vi "Sub_Initialize_LEMP_del.vi"(1 "Stiff":T2, 2 "Mass":T2) -> (0 "LEMP":T1)   [LabVIEW 2021]
uses:
  <vilib>/Analysis/Matrix/Datatypes/RealMatrix.ctl
  <vilib>/Analysis/Matrix/Numeric/Conversions/Matrix To Array - RM.vi
  <vilib>/Analysis/Matrix/NI_Matrix.lvlib
panel:
  # "Input"
  # "Output"
  # "This VI acquires the required input cluster for the Sub_online_LEMP_Update.vi, this VI calls on SciPy.linalg.eigh() due to issues with the standard \"General Eigenvalues and Eigenvectors.vi\" outputting inappropriately scaled eigenvectors for the LEMP. Additionally the Bitedness of this installation of LabVIEW does not match with Python so direct python calls were similarly unavailable. The workaround involved a saving the matrices in a text format command line calling the SciPy eigh function saving that output as a text file, then load the output file in to memory (See Sub_Python_cmd_eigh.vi, getEigenCommandPrompt.py , mass.lvm, stiff.lvm,eigenvalues.txt, eigenvectors.txt).\n\n              - Alexander Vereen AFRL Summer scholars 2022"
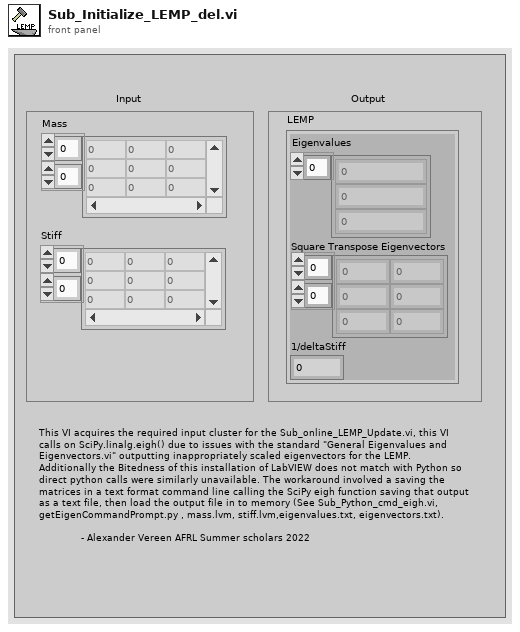
[diagram p1: front panel]
types:
  T1 = cluster{"Eigenvalues":dbl[], "Square Transpose Eigenvectors":dbl[][], "1/deltaStiff":dbl}
  T2 = typedef "NI_Matrix.lvlib/RealMatrix.ctl" = dbl[][]
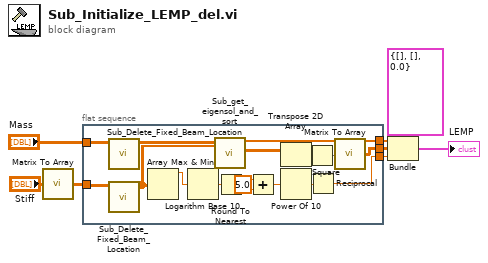
[diagram p0: block diagram]
diagram:
  n1 = call-poly <vilib>:"Matrix To Array.vi"("Real Matrix"="Stiff") -> ("Real 2D Array"=w7:dbl[][])
  n2 = flat-sequence {
    tunnel: [w23] -> w4
    tunnel: [w19] -> w3
    tunnel: [w20] -> w2
    tunnel: "Mass" -> [w18]
    tunnel: w7 -> [w16]
    frame #0 {
      n3 = call "Sub_Delete_Fixed_Beam_Location.vi"("Pre-BC Matrix"=w18) -> ("Post-BC Matrix"=w17:dbl[][])  [unwired: 10 in]
      n4 = call "Sub_Delete_Fixed_Beam_Location.vi"("Pre-BC Matrix"=w16) -> ("Post-BC Matrix"=w15:dbl[][])  [unwired: 10 in]
      n5 = Array Max & Min(array=w15) -> (max value=w9:dbl)  [unwired: 3 out]
      n6 = Logarithm Base 10(1:w9) -> (0:w12:dbl)
      n7 = call "Sub_get_eigensol_and_sort.vi"("Mass"=w17, "Stiffness"=w15) -> ("Unsorted Eigenvalues"=w23:dbl[], "Unsorted Eigenvector Matrix"=w22:T2)  [unwired: 13 in, 3 out]
      n8 = Round To Nearest(number=w12) -> (nearest integer value=w13:dbl)
      n9 = Add(x=w13, y=5.0) -> (x+y=w14:dbl)
      n10 = Transpose 2D Array(2D array=w22) -> (transposed array=w24:T2)
      n11 = Power Of 10(x=w14) -> (10^x=w10:dbl)
      n12 = Square(x=w24) -> (x^2=w21:T2)
      n13 = Reciprocal(x=w10) -> (1/x=w20:dbl)
      n14 = call-poly <vilib>:"Matrix To Array.vi"("Real Matrix"=w21) -> ("Real 2D Array"=w19:dbl[][])
    }
  }
  n15 = Bundle(cluster=T1 {"Eigenvalues"=[], "Square Transpose Eigenvectors"=[], "1/deltaStiff"=0.0} ("LEMP"), "Eigenvalues"=w4, "Square Transpose Eigenvectors"=w3, "1/deltaStiff"=w2) -> (→"LEMP":T1)
